vi "Core.vi"(8 "error in (no error)":errorcluster, 11 "TCP in":refnum<class "TCP.lvclass">) -> (0 "error out":errorcluster, 3 "TCP out":refnum<class "TCP.lvclass">)   [LabVIEW 2021, in "TCP.lvclass"]
uses:
  TCP.lvclass
  D:/my_projects/projects/Algorithms/Labview/21/Master CR/Master CR.lvclass
  ctl/CR_Core_State.ctl
  Master CR.lvclass/Master CR.ctl
  Status/Run/Write Run.vi
  Status/write/Write write.vi
  Modbus_v121c/Data Model/Device Data Model.lvclass
  TCP.lvclass/TCP.ctl
  Master CR.lvclass
panel:
  out "MB_TCP_State":T1=enum."requests"
  in  "write enable":bool=TRUE
  in  "stop":bool
  out "stopped":bool
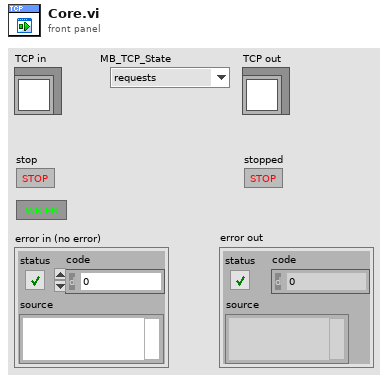
[diagram p1: front panel]
types:
  T1 = typedef "Master CR.lvclass/CR_Core_State.ctl" = enum8{"initialization", "redefine", "standby", "ping", "connect", "wait to reconnect", "wait to reset timeout", "configure", "requests", "close connection", "stop"}
  T2 = typedef "Master CR.lvclass/MB timeouts.ctl" = cluster{"reconn_timeout":i32, "N attempt max":i32, "t_reset_TTL":i32, "period":i32}
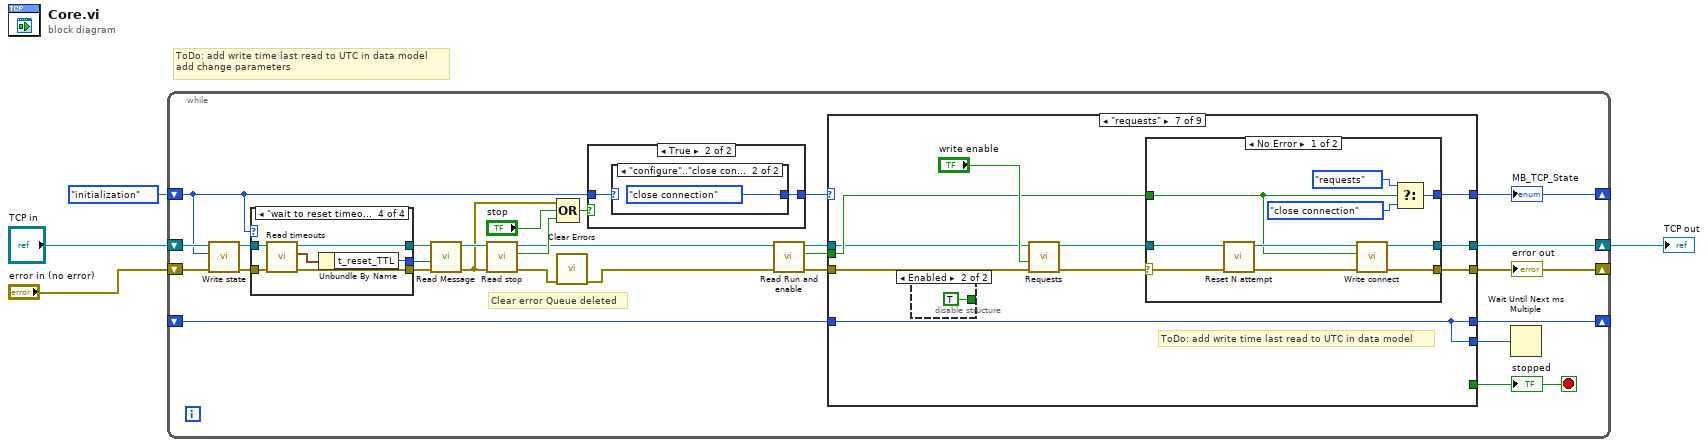
[diagram p0: block diagram]
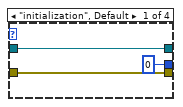
[diagram p2: hidden frame]
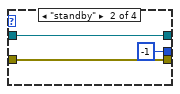
[diagram p3: hidden frame]
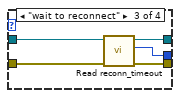
[diagram p4: hidden frame]
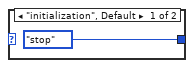
[diagram p6: hidden frame]
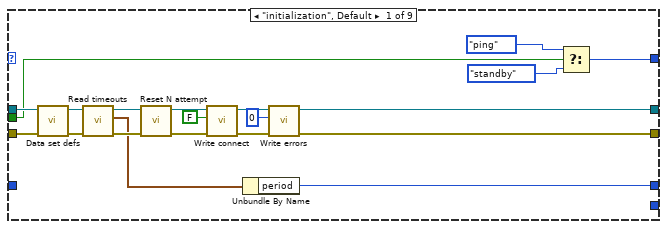
[diagram p7: hidden frame]
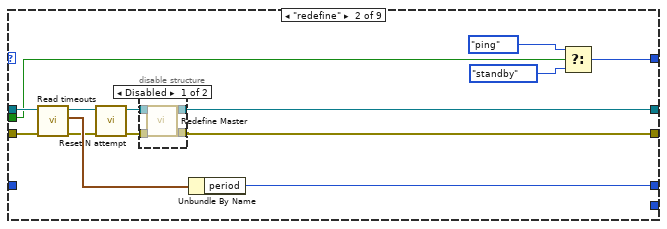
[diagram p8: hidden frame]
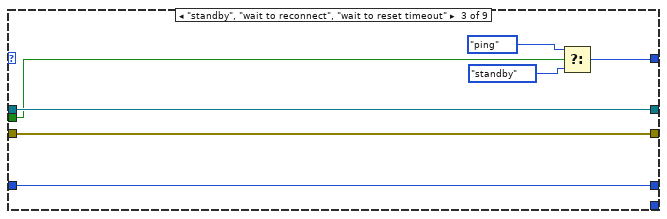
[diagram p10: hidden frame]
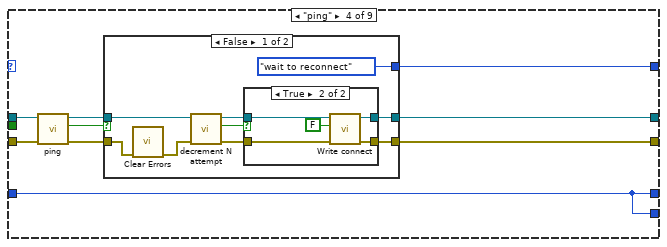
[diagram p11: hidden frame]
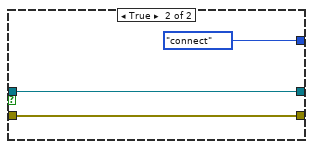
[diagram p13: hidden frame]
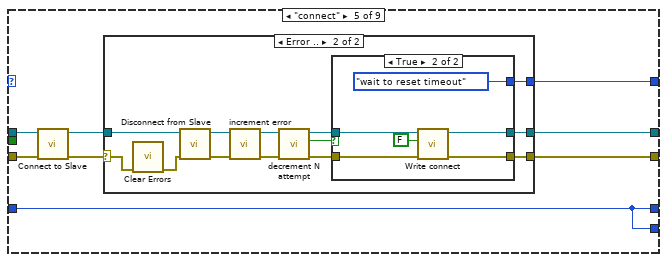
[diagram p14: hidden frame]
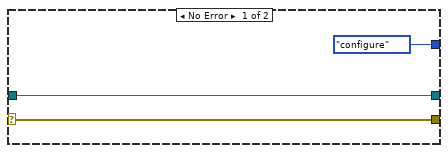
[diagram p15: hidden frame]
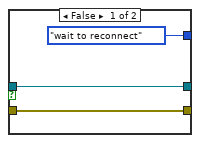
[diagram p16: hidden frame]
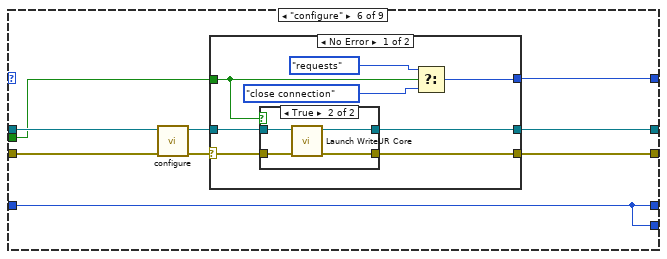
[diagram p17: hidden frame]
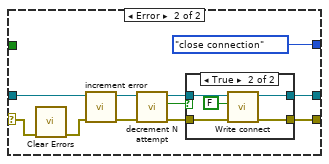
[diagram p19: hidden frame]
diagram:
  # "ToDo: add write time last read to UTC in data model\nadd change parameters"
  n1 = while {
    shift-right: [w28] -> w4
    shift-left: "TCP in" -> [w11]
    shift-right: [w24] -> _
    shift-left: "error in (no error)" -> [w10]
    shift-right: [w30] -> _
    shift-left: _ -> [w31]
    shift-right: [w25] -> _
    shift-left: CR_Core_State."initialization" ("state") -> [w9]
    stop <- w23 stop-if-true
    # "Clear error Queue deleted"
    n2 = call "Write state.vi"("error in (no error)"=w10, "state"=w9, "Master CR in"=w11) -> ("error out"=w16:errorcluster, "Master CR out"=w15:refnum<class "TCP.lvclass">)  [unwired: 7 in]
    n3 = case shown="\"wait to reset timeout\"" w9 {
      tunnel: w15 -> [w33 w36 w42 w47]
      tunnel: w16 -> [w32 w35 w41 w46]
      tunnel: [w33 w36 w40 w45] -> w12
      tunnel: [w32 w35 w39 w44] -> w13
      tunnel: [0 ("timeout (0)") -1 ("timeout (0)") w38 w43] -> w14
      frame "initialization", Default {
      }
      frame "standby" {
      }
      frame "wait to reconnect" {
        n4 = call "Read reconn_timeout.vi"("error in (no error)"=w41, "Master CR in"=w42) -> ("error out"=w39:errorcluster, "reconn_timeout"=w38:i32, "Master CR out"=w40:refnum<class "TCP.lvclass">)  [unwired: 7 in]
      }
      frame "wait to reset timeout" {
        n5 = call "Read timeouts.vi"("error in (no error)"=w46, "Master CR in"=w47) -> ("error out"=w44:errorcluster, "MB timeouts"=w48:T2, "Master CR out"=w45:refnum<class "TCP.lvclass">)  [unwired: 7 in]
        n6 = Unbundle By Name(w48) -> ("t_reset_TTL"=w43:i32)
      }
    }
    n7 = call "Read Message.vi"("error in (no error)"=w13, "timeout (0)"=w14, "Master CR in"=w12) -> ("error out"=w7:errorcluster, "Master CR out"=w8:refnum<class "TCP.lvclass">)  [unwired: 6 in, 1 out]
    n8 = call "Read stop.vi"("error in (no error)"=w7, "Master CR in"=w8) -> ("error out"=w6:errorcluster, "Stop"=w22:bool, "Master CR out"=w21:refnum<class "TCP.lvclass">)  [unwired: 7 in]
    n9 = Compound Arithmetic op=OR(w7, "stop", w22) -> (w26:bool)
    n10 = call <vilib>:"Clear Errors.vi"("error in (no error)"=w6) -> ("error out"=w5:errorcluster)  [unwired: 5 in, 1 out]
    n11 = case shown="True" w26 {
      tunnel: w9 -> [w49 w51]
      tunnel: [w49 w50] -> w27
      frame False {
      }
      frame True {
        n12 = case shown="\"configure\"..\"close connection\"" w51 {
          tunnel: [CR_Core_State."stop" ("MB_TCP_State") CR_Core_State."close connection" ("MB_TCP_State")] -> w50
          frame "initialization", Default {
          }
          frame "configure".."close connection" {
          }
        }
      }
    }
    n13 = call "Read Run and enable.vi"("error in (no error)"=w5, "Master CR in"=w21) -> ("error out"=w20:errorcluster, "Enable and Run"=w18:bool, "Master CR out"=w19:refnum<class "TCP.lvclass">)  [unwired: 7 in]
    n14 = case shown="\"requests\"" w27 {
      tunnel: [_ _ _ _ _ _ _ _ TRUE] -> w23
      tunnel: w19 -> [w71 w84 w96 w105 w132 w164 w203 w252 w259]
      tunnel: [w56 w76 w96 w109 w136 w170 w211 w243 w262] -> w28
      tunnel: w20 -> [w72 w83 w95 w104 w133 w162 w202 w251 w258]
      tunnel: [w57 w85 w97 w108 w135 w169 w210 w245 CR_Core_State."initialization" ("MB_TCP_State")] -> w25
      tunnel: [w55 w75 w95 w107 w134 w168 w209 w242 w261] -> w24
      tunnel: [w73 w81 w100 w106 w129 w167 w207 w253 w266] -> w30
      tunnel: w31 -> [_ _ w100 w106 w129 w167 w207 w253 w266]
      tunnel: [_ _ _ w106 w129 w167 w207 _ _] -> w29
      tunnel: w18 -> [w54 w74 w94 _ _ w163 w204 w244 _]
      frame "initialization", Default {
        n15 = call "Data set defs.vi"("error in (no error)"=w72, "Master CR in"=w71) -> ("error out"=w66:errorcluster, "Master CR out"=w69:refnum<class "TCP.lvclass">)  [unwired: 8 in]
        n16 = call "Read timeouts.vi"("error in (no error)"=w66, "Master CR in"=w69) -> ("error out"=w70:errorcluster, "MB timeouts"=w67:T2, "Master CR out"=w68:refnum<class "TCP.lvclass">)  [unwired: 7 in]
        n17 = call "Reset N attempt.vi"("error in (no error)"=w70, "Master CR in"=w68) -> ("error out"=w64:errorcluster, "Master CR out"=w65:refnum<class "TCP.lvclass">)  [unwired: 8 in]
        n18 = call "Write connect.vi"("error in (no error)"=w64, "connect"=FALSE, "Master CR in"=w65) -> ("error out"=w62:errorcluster, "Master CR out"=w61:refnum<class "TCP.lvclass">)  [unwired: 7 in]
        n19 = Unbundle By Name(w67) -> ("period"=w73:i32)
        n20 = call "Write errors.vi"("error in (no error)"=w62, "errors"=0, "Master CR in"=w61) -> ("error out"=w55:errorcluster, "Master CR out"=w56:refnum<class "TCP.lvclass">)  [unwired: 7 in]
        n21 = Select(t=CR_Core_State."ping" ("MB_TCP_State"), s=w54, f=CR_Core_State."standby" ("MB_TCP_State")) -> (s? t:f=w57:T1)
      }
      frame "redefine" {
        n22 = call "Read timeouts.vi"("error in (no error)"=w83, "Master CR in"=w84) -> ("error out"=w80:errorcluster, "MB timeouts"=w82:T2, "Master CR out"=w79:refnum<class "TCP.lvclass">)  [unwired: 7 in]
        n23 = call "Reset N attempt.vi"("error in (no error)"=w80, "Master CR in"=w79) -> ("error out"=w77:errorcluster, "Master CR out"=w78:refnum<class "TCP.lvclass">)  [unwired: 8 in]
        n24 = disable-structure shown="Disabled" {
          disable-tunnel: w78 -> [w91 w93]
          disable-tunnel: w77 -> [w90 w92]
          disable-tunnel: [w89 w93] -> w76
          disable-tunnel: [w88 w92] -> w75
          frame Disabled {
            n25 = call "Redefine Master.vi"("error in (no error)"=w90, "Master CR in"=w91) -> ("error out"=w88:errorcluster, "Master CR out"=w89:refnum<class "TCP.lvclass">)  [unwired: 8 in]
          }
          frame Enabled {
          }
        }
        n26 = Unbundle By Name(w82) -> ("period"=w81:i32)
        n27 = Select(t=CR_Core_State."ping" ("MB_TCP_State"), s=w74, f=CR_Core_State."standby" ("MB_TCP_State")) -> (s? t:f=w85:T1)
      }
      frame "standby", "wait to reconnect", "wait to reset timeout" {
        n28 = Select(t=CR_Core_State."ping" ("MB_TCP_State"), s=w94, f=CR_Core_State."standby" ("MB_TCP_State")) -> (s? t:f=w97:T1)
      }
      frame "ping" {
        n29 = call-dynamic "ping.vi"("error in (no error)"=w104, "TCP in"=w105) -> ("error out"=w101:errorcluster, "Ping OK"=w102:bool, "TCP out"=w103:refnum<class "TCP.lvclass">)  [unwired: 7 in]
        n30 = case shown="False" w102 {
          tunnel: w103 -> [w112 w128]
          tunnel: [CR_Core_State."wait to reconnect" ("MB_TCP_State") CR_Core_State."connect" ("MB_TCP_State")] -> w108
          tunnel: [w117 w128] -> w109
          tunnel: [w116 w126] -> w107
          tunnel: w101 -> [w113 w126]
          frame False {
            n31 = call <vilib>:"Clear Errors.vi"("error in (no error)"=w113) -> ("error out"=w111:errorcluster)  [unwired: 5 in, 1 out]
            n32 = call "decrement N attempt.vi"("error in (no error)"=w111, "Master CR in"=w112) -> ("error out"=w114:errorcluster, "=0"=w118:bool, "Master CR out"=w115:refnum<class "TCP.lvclass">)  [unwired: 7 in]
            n33 = case shown="True" w118 {
              tunnel: w115 -> [w120 w122]
              tunnel: [w120 w125] -> w117
              tunnel: w114 -> [w119 w121]
              tunnel: [w119 w123] -> w116
              frame False {
              }
              frame True {
                n34 = call "Write connect.vi"("error in (no error)"=w121, "connect"=FALSE, "Master CR in"=w122) -> ("error out"=w123:errorcluster, "Master CR out"=w125:refnum<class "TCP.lvclass">)  [unwired: 7 in]
              }
            }
          }
          frame True {
          }
        }
      }
      frame "connect" {
        n35 = call-dynamic "Connect to Slave.vi"("error in (no error)"=w133, "TCP master in"=w132) -> ("error out"=w130:errorcluster, "TCP master out"=w131:refnum<class "TCP.lvclass">)  [unwired: 8 in]
        n36 = case shown="Error .." w130 {
          selector: w130 -> [w137 w144]
          tunnel: w131 -> [w138 w145]
          tunnel: [CR_Core_State."configure" ("MB_TCP_State") w150] -> w135
          tunnel: [w138 w149] -> w136
          tunnel: [w137 w148] -> w134
          frame No Error {
          }
          frame Error {
            n37 = call <vilib>:"Clear Errors.vi"("error in (no error)"=w144) -> ("error out"=w143:errorcluster)  [unwired: 5 in, 1 out]
            n38 = call-dynamic "Disconnect from Slave.vi"("error in"=w143, "TCP master in"=w145) -> ("error out"=w146:errorcluster, "TCP master out"=w147:refnum<class "TCP.lvclass">)  [unwired: 8 in]
            n39 = call "increment error.vi"("error in (no error)"=w146, "Master CR in"=w147) -> ("error out"=w142:errorcluster, "Master CR out"=w152:refnum<class "TCP.lvclass">)  [unwired: 7 in, 1 out]
            n40 = call "decrement N attempt.vi"("error in (no error)"=w142, "Master CR in"=w152) -> ("error out"=w140:errorcluster, "=0"=w151:bool, "Master CR out"=w141:refnum<class "TCP.lvclass">)  [unwired: 7 in]
            n41 = case shown="True" w151 {
              tunnel: [CR_Core_State."wait to reconnect" ("MB_TCP_State") CR_Core_State."wait to reset timeout" ("MB_TCP_State")] -> w150
              tunnel: w141 -> [w154 w157]
              tunnel: [w154 w160] -> w149
              tunnel: w140 -> [w153 w156]
              tunnel: [w153 w158] -> w148
              frame False {
              }
              frame True {
                n42 = call "Write connect.vi"("error in (no error)"=w156, "connect"=FALSE, "Master CR in"=w157) -> ("error out"=w158:errorcluster, "Master CR out"=w160:refnum<class "TCP.lvclass">)  [unwired: 7 in]
              }
            }
          }
        }
      }
      frame "configure" {
        n43 = call-dynamic "configure.vi"("error in (no error)"=w162, "Master CR in"=w164) -> ("error out"=w165:errorcluster, "Master CR out"=w166:refnum<class "TCP.lvclass">)  [unwired: 8 in]
        n44 = case shown="No Error" w165 {
          selector: w165 -> [w174 w193]
          tunnel: [w178 CR_Core_State."close connection" ("MB_TCP_State")] -> w169
          tunnel: [w172 w186] -> w168
          tunnel: w166 -> [w175 w185]
          tunnel: [w173 w187] -> w170
          tunnel: w163 -> [w171 _]
          frame No Error {
            n45 = case shown="True" w171 {
              tunnel: w175 -> [w180 w181]
              tunnel: w174 -> [w179 w183]
              tunnel: [w179 w182] -> w172
              tunnel: [w180 w181] -> w173
              frame False {
              }
              frame True {
                n46 = call "Launch WriteUR Core.vi"("error in"=w183, "Master CR in"=w181) -> ("error out"=w182:errorcluster)  [unwired: 9 in]
              }
            }
            n47 = Select(t=CR_Core_State."requests" ("MB_TCP_State"), s=w171, f=CR_Core_State."close connection" ("MB_TCP_State")) -> (s? t:f=w178:T1)
          }
          frame Error {
            n48 = call <vilib>:"Clear Errors.vi"("error in (no error)"=w193) -> ("error out"=w184:errorcluster)  [unwired: 5 in, 1 out]
            n49 = call "increment error.vi"("error in (no error)"=w184, "Master CR in"=w185) -> ("error out"=w189:errorcluster, "Master CR out"=w188:refnum<class "TCP.lvclass">)  [unwired: 7 in, 1 out]
            n50 = call "decrement N attempt.vi"("error in (no error)"=w189, "Master CR in"=w188) -> ("error out"=w190:errorcluster, "=0"=w192:bool, "Master CR out"=w191:refnum<class "TCP.lvclass">)  [unwired: 7 in]
            n51 = case shown="True" w192 {
              tunnel: w191 -> [w196 w201]
              tunnel: [w196 w200] -> w187
              tunnel: w190 -> [w195 w199]
              tunnel: [w195 w197] -> w186
              frame False {
              }
              frame True {
                n52 = call "Write connect.vi"("error in (no error)"=w199, "connect"=FALSE, "Master CR in"=w201) -> ("error out"=w197:errorcluster, "Master CR out"=w200:refnum<class "TCP.lvclass">)  [unwired: 7 in]
              }
            }
          }
        }
      }
      frame "requests" {
        # "ToDo: add write time last read to UTC in data model"
        n53 = disable-structure shown="Enabled" {
          disable-tunnel: [w212 TRUE] -> _
          frame Disabled {
            n54 = Equal?() -> (x = y?=w212:bool)  [unwired: 2 in]
          }
          frame Enabled {
          }
        }
        n55 = call-dynamic "Requests.vi"("error in (no error)"=w202, "write enable"="write enable", "TCP in"=w203) -> ("error out"=w206:errorcluster, "TCP out"=w208:refnum<class "TCP.lvclass">)  [unwired: 7 in]
        n56 = case shown="No Error" w206 {
          selector: w206 -> [w219 w234]
          tunnel: [w223 CR_Core_State."close connection" ("MB_TCP_State")] -> w210
          tunnel: w204 -> [w216 _]
          tunnel: [w214 w230] -> w209
          tunnel: w208 -> [w220 w227]
          tunnel: [w217 w231] -> w211
          frame No Error {
            n57 = call "Reset N attempt.vi"("error in (no error)"=w219, "Master CR in"=w220) -> ("error out"=w215:errorcluster, "Master CR out"=w218:refnum<class "TCP.lvclass">)  [unwired: 8 in]
            n58 = call "Write connect.vi"("error in (no error)"=w215, "connect"=w216, "Master CR in"=w218) -> ("error out"=w214:errorcluster, "Master CR out"=w217:refnum<class "TCP.lvclass">)  [unwired: 7 in]
            n59 = Select(t=CR_Core_State."requests" ("MB_TCP_State"), s=w216, f=CR_Core_State."close connection" ("MB_TCP_State")) -> (s? t:f=w223:T1)
          }
          frame Error {
            # "clear read error"
            n60 = call <vilib>:"Clear Errors.vi"("error in (no error)"=w234) -> ("error out"=w226:errorcluster)  [unwired: 5 in, 1 out]
            n61 = call "increment error.vi"("error in (no error)"=w226, "Master CR in"=w227) -> ("error out"=w228:errorcluster, "Master CR out"=w233:refnum<class "TCP.lvclass">)  [unwired: 7 in, 1 out]
            n62 = call "decrement N attempt.vi"("error in (no error)"=w228, "Master CR in"=w233) -> ("error out"=w229:errorcluster, "=0"=w225:bool, "Master CR out"=w232:refnum<class "TCP.lvclass">)  [unwired: 7 in]
            n63 = case shown="False" w225 {
              tunnel: w232 -> [w236 w241]
              tunnel: [w236 w240] -> w231
              tunnel: w229 -> [w235 w239]
              tunnel: [w235 w237] -> w230
              frame False {
              }
              frame True {
                n64 = call "Write connect.vi"("error in (no error)"=w239, "connect"=FALSE, "Master CR in"=w241) -> ("error out"=w237:errorcluster, "Master CR out"=w240:refnum<class "TCP.lvclass">)  [unwired: 7 in]
              }
            }
          }
        }
      }
      frame "close connection" {
        n65 = call-dynamic "Disconnect from Slave.vi"("error in"=w251, "TCP master in"=w252) -> ("error out"=w242:errorcluster, "TCP master out"=w243:refnum<class "TCP.lvclass">)  [unwired: 8 in]
        n66 = disable-structure shown="Enabled" {
          disable-tunnel: [w254 TRUE] -> w246
          frame Disabled {
            n67 = Equal?() -> (x = y?=w254:bool)  [unwired: 2 in]
          }
          frame Enabled {
          }
        }
        n68 = Select(t=CR_Core_State."wait to reconnect" ("MB_TCP_State"), s=w246, f=CR_Core_State."redefine" ("MB_TCP_State")) -> (s? t:f=w248:T1)
        n69 = Select(t=w248, s=w244, f=CR_Core_State."standby" ("MB_TCP_State")) -> (s? t:f=w245:T1)
      }
      frame "stop" {
        n70 = call "Write connect.vi"("error in (no error)"=w258, "connect"=FALSE, "Master CR in"=w259) -> ("error out"=w257:errorcluster, "Master CR out"=w260:refnum<class "TCP.lvclass">)  [unwired: 7 in]
        n71 = call "Write stop.vi"("error in (no error)"=w257, "Stop"=FALSE, "Master CR in"=w260) -> ("error out"=w261:errorcluster, "Master CR out"=w262:refnum<class "TCP.lvclass">)  [unwired: 7 in]
      }
    }
    "stopped" <- w23
    "error out" <- w24
    "MB_TCP_State" <- w25
    n72 = Wait Until Next ms Multiple(millisecond multiple=w29) -> ()  [unwired: 1 out]
  }
  "TCP out" <- w4
